vi "LVDT-FFT.vi"() -> ()   [LabVIEW 2011]
uses:
  <vilib>/Platform/TimedLoop/XDataNode/timing_clust.ctl
  <vilib>/Platform/TimedLoop/XDataNode/nitl_modes.ctl
  <vilib>/Platform/TimedLoop/XDataNode/wakeup.ctl
  <vilib>/Analysis/2dsp.llb/Real FFT.vi
  <vilib>/Platform/TimedLoop/XDataNode/XDataNode.xnode
  <vilib>/Analysis/NI_AALPro.lvlib
  <vilib>/Platform/TimedLoop/XDataNode/XDNodeRunTimeDep.lvlib
panel:
  in  "Simulation":bool
  in  "FTT-samples":i32=1000
  in  "Level":dbl
  in  "Frequency":dbl
  in  "Remove DC":bool
  in  "DC Level":bool
  in  "Sinus":bool
  in  "Random":bool
  in  "stop":bool
  out "FFT graph":dbl[](graph)
  out "FFT {X}":dbl[](array[numeric])
  out "Time Series":cluster{dbl, dbl, dbl[]}(graph)
  in  "Slide":dbl(slide) scale=0.0..25.0
  in  "n_sample":i32
  out "Complete Data":dbl[](array[numeric])
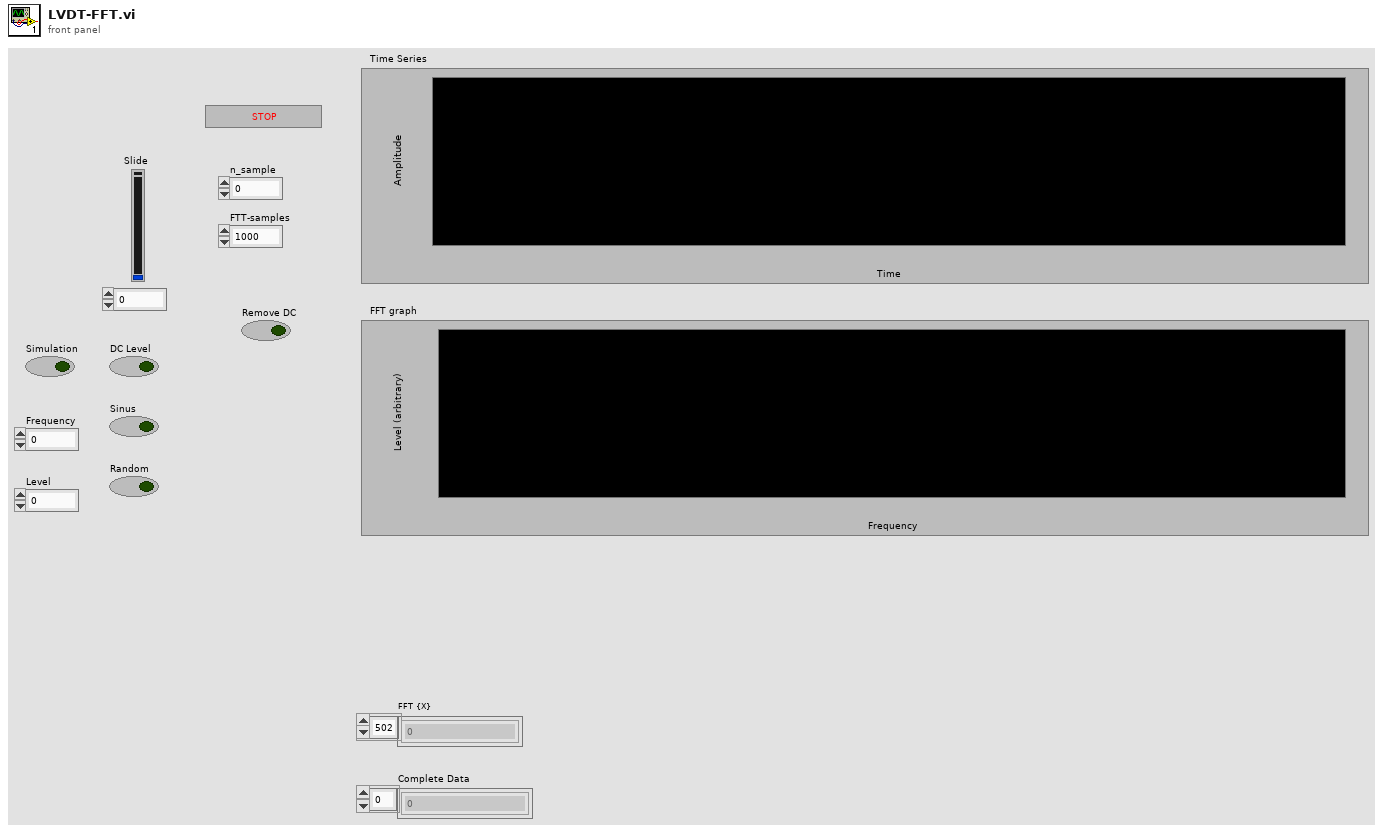
[diagram p1: front panel]
types:
  T1 = typedef "XDNodeRunTimeDep.lvlib/timing_clust.ctl" = cluster{"Expected End [f-1]":u64, "Actual End [f-1]":u64, "Finished Late? [f-1]":bool, "Expected End [i-1]":u64, "Actual End [i-1]":u64, "Finished Late? [i-1]":bool, "Expected Start [i]":u64, "Actual Start [i]":u64, "Expected Start [f]":u64, "Actual Start [f]":u64, "Source Name":string, "Structure Name":string, "Period":i64, "Deadline":i64, "Offset":i64, "Start":i64, "Priority":i32, "Timeout":i32, "Mode":T2, "Wakeup Reason":T3, "Error":errorcluster, "Source Type":string, "Secondary Source Type":string, "Global End Time":u64, "Global Start Time":u64, "Frame Duration":u64, "Iteration Duration":u64, "Assigned CPU":i32, "I/O Scan Engine Mode":u32}
  T2 = typedef "XDNodeRunTimeDep.lvlib/nitl_modes.ctl" = enum32{"No Change", "Process missed periods, maintain original phase", "Discard missed periods, maintain original phase", "Process missed periods, ignore original phase", "Discard missed periods, ignore original phase"}
  T3 = typedef "XDNodeRunTimeDep.lvlib/wakeup.ctl" = enum32{"Normal", "Aborted", "Asynchronous wakeup", "Timing source error", "Timed loop error", "Timeout"}
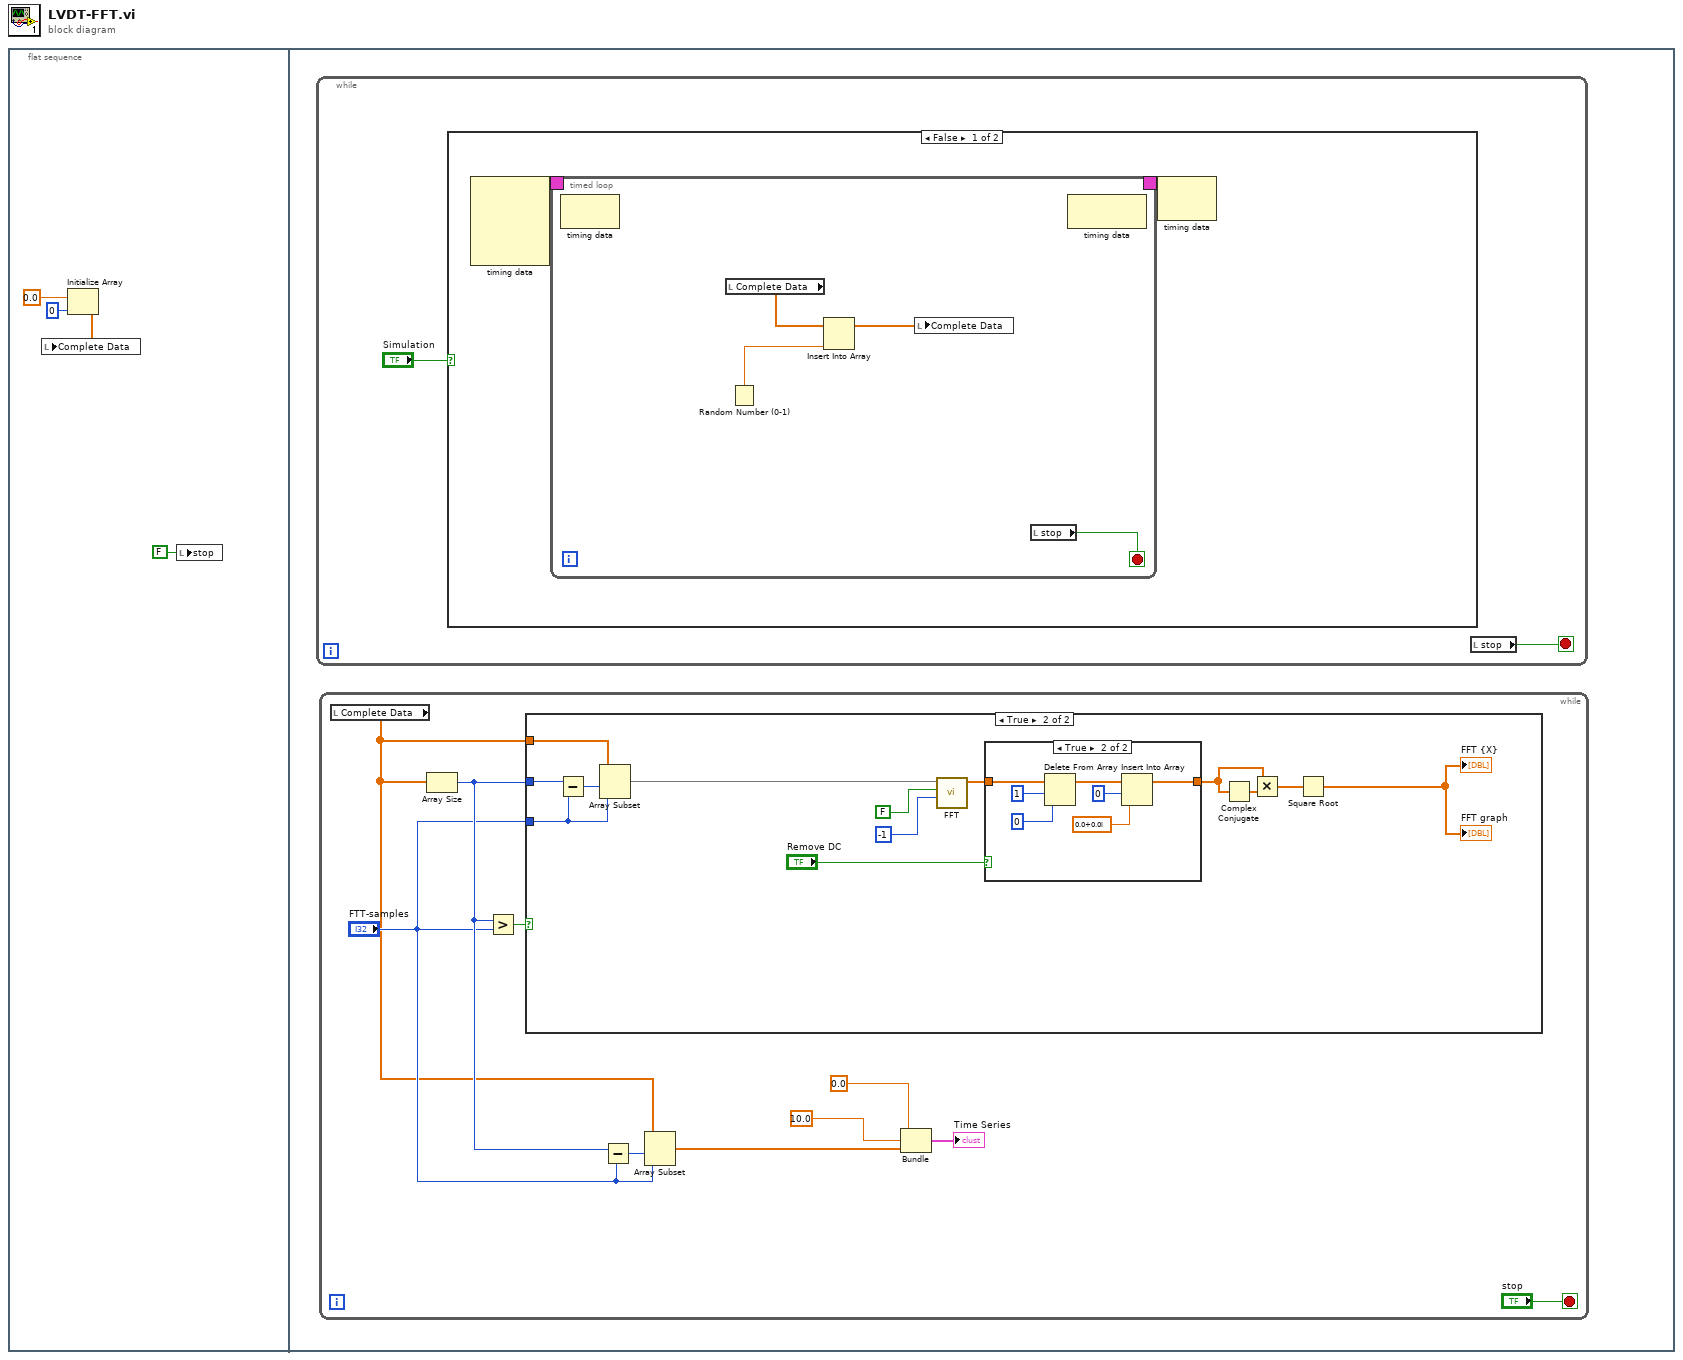
[diagram p0: block diagram]
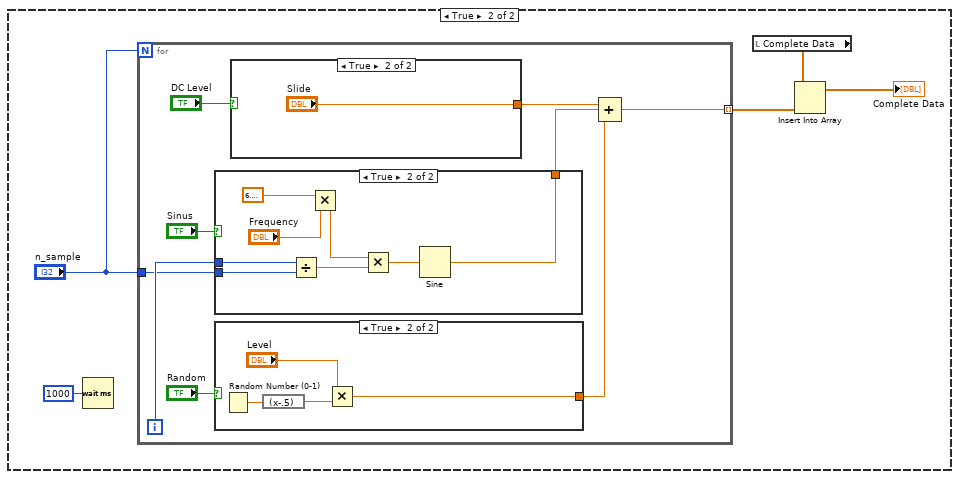
[diagram p2: hidden frame]
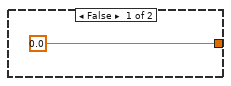
[diagram p3: hidden frame]
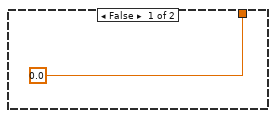
[diagram p4: hidden frame]
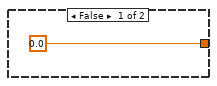
[diagram p5: hidden frame]
diagram:
  n1 = flat-sequence {
    frame #0 {
      n2 = Initialize Array(0.0, 0 ("dimension size")) -> (w2:dbl[])
      n3 = local write "Complete Data"(w2) -> ()
      n4 = local write "stop"(FALSE ("stop")) -> ()
    }
    frame #1 {
      n5 = while {
        stop <- w6 stop-if-true
        n6 = case shown="False" "Simulation" {
          frame False {
            n7 = node-c288() -> (w8:T1)  [unwired: 4 in]
            n8 = timed-loop {
              timing: w8 -> [_]
              timing-out: [_] -> w7
              stop <- w9 stop-if-true
              n9 = node-c288() -> ()  [unwired: 1 in, 1 out]
              n10 = local read "Complete Data"() -> (w11:dbl[])
              n11 = Random Number (0-1)() -> (number: 0 to 1=w10:dbl)
              n12 = Insert Into Array(array=w11, new element=w10) -> (w12:dbl[])  [unwired: 1 in]
              n13 = local write "Complete Data"(w12) -> ()
              n14 = local read "stop"() -> (w9:bool)
              n15 = node-c288() -> ()  [unwired: 1 in, 1 out]
            }
            n16 = node-c288(w7) -> ()  [unwired: 1 out]
          }
          frame True {
            n17 = Wait (ms)(milliseconds to wait=u32 1000) -> ()  [unwired: 1 out]
            n18 = for {
              N: "n_sample" -> [_]
              tunnel: [w30] -> w18 mode=indexing
              tunnel: "n_sample" -> [w25]
              i -> [w26]
              n19 = case shown="True" "Sinus" {
                tunnel: [0.0 ("number: 0 to 1") w41] -> w28
                tunnel: w26 -> [_ w40]
                tunnel: w25 -> [_ w39]
                frame False {
                }
                frame True {
                  n20 = Divide(x=w40, y=w39) -> (x/y=w38:dbl)
                  n21 = Multiply(x=6.283185307179586, y="Frequency") -> (x*y=w36:dbl)
                  n22 = Multiply(x=w36, y=w38) -> (x*y=w37:dbl)
                  n23 = Sine(x=w37) -> (sin(x)=w41:dbl)
                }
              }
              n24 = case shown="True" "Random" {
                tunnel: [0.0 ("number: 0 to 1") w44] -> w29
                frame False {
                }
                frame True {
                  n25 = Random Number (0-1)() -> (number: 0 to 1=w46:dbl)
                  n26 = expression code="(x-.5)"(w46) -> (w45:dbl)
                  n27 = Multiply(x="Level", y=w45) -> (x*y=w44:dbl)
                }
              }
              n28 = case shown="True" "DC Level" {
                tunnel: [0.0 ("number: 0 to 1") "Slide"] -> w27
                frame False {
                }
                frame True {
                }
              }
              n29 = Compound Arithmetic op=ADD(w27, w28, w29) -> (w30:dbl)
            }
            n30 = local read "Complete Data"() -> (w20:dbl[])
            n31 = Insert Into Array(array=w20, new element=w18) -> (→"Complete Data":dbl[])  [unwired: 1 in]
          }
        }
        n32 = local read "stop"() -> (w6:bool)
      }
      n33 = while {
        stop <- "stop" stop-if-true
        n34 = local read "Complete Data"() -> (w47:dbl[])
        n35 = Array Size(array=w47) -> (size(s)=w53:i32)
        n36 = Greater?(x=w53, y="FTT-samples") -> (0:w55:bool)
        n37 = case shown="True" w55 {
          tunnel: "FTT-samples" -> [_ w65]
          tunnel: w53 -> [_ w67]
          tunnel: w47 -> [_ w57]
          frame False {
          }
          frame True {
            n38 = Subtract(x=w67, y=w65) -> (x-y=w66:i32)
            n39 = Array Subset(array=w57, index=w66, length=w65) -> (w58:dbl[])
            n40 = call-poly <vilib>:"FFT.vi"("FFT size"=-1, "shift?"=FALSE, "X"=w58) -> ("FFT {X}"=w63:cdb[])  [unwired: 7 in, 1 out]
            n41 = case shown="True" "Remove DC" {
              tunnel: w63 -> [w70 w77]
              tunnel: [w70 w73] -> w62
              frame False {
              }
              frame True {
                n42 = Delete From Array(array=w77, length=1, index=0 ("FFT size")) -> (array with subset deleted=w74:cdb[])  [unwired: 1 out]
                n43 = Insert Into Array(array=w74, index=0 ("FFT size"), new element=cdb 0.0+0.0i ("new element/subarray")) -> (w73:cdb[])
              }
            }
            n44 = Complex Conjugate(1:w62) -> (0:w64:cdb[])
            n45 = Multiply(x=w62, y=w64) -> (x*y=w60:cdb[])
            n46 = Square Root(x=w60) -> (sqrt(x)=→"FFT {X}" →"FFT graph":cdb[])
          }
        }
        n47 = Subtract(x=w53, y="FTT-samples") -> (x-y=w54:i32)
        n48 = Array Subset(array=w47, index=w54, length="FTT-samples") -> (w48:dbl[])
        n49 = Bundle(0.0, 10.0, w48) -> (→"Time Series":cluster{dbl, dbl, dbl[]})  [unwired: 1 in]
      }
    }
  }
